vi "calibrationSpectrometer_issueCommand_ExitControl.vi"(8 "error in (no error)":errorcluster, 11 "command_ExitControl_Ctl":T1) -> (0 "error out":errorcluster, 2 "function return":i32, 3 "command_ExitControl_Ctl out":T1)   [LabVIEW 2016, in "SALLV_calibrationSpectrometer.lvlib"]
doc: "int calibrationSpectrometer_shm_issueCommand_ExitControlLV(calibrationSpectrometer_command_ExitControlLV *command_ExitControl_Ctl );"
uses:
  SALLV_calibrationSpectrometer.lvlib
  DataTypes/command_ExitControl.ctl
  SALLV_calibrationSpectrometer.so
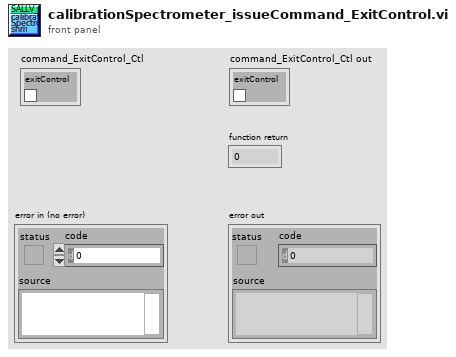
[diagram p1: front panel]
types:
  T1 = typedef "SALLV_calibrationSpectrometer.lvlib/command_ExitControl.ctl" = cluster{"exitControl":bool}
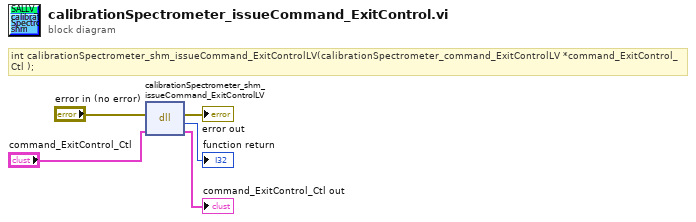
[diagram p0: block diagram]
diagram:
  # "int calibrationSpectrometer_shm_issueCommand_ExitControlLV(calibrationSpectrometer_command_ExitControlLV *command_ExitControl_Ctl );"
  n1 = dll-call lib="home/harini/TCS/sallv_sedspectrometer/SALLV_calibrationSpectrometer.*" fn="calibrationSpectrometer_shm_issueCommand_ExitControlLV"(error in="error in (no error)", "command_ExitControl_Ctl"="command_ExitControl_Ctl") -> (error out=→"error out":errorcluster, →"function return":i32, "command_ExitControl_Ctl"=→"command_ExitControl_Ctl out":T1)  [unwired: 2 in, 1 out]
